vi "Trawnik.vi"() -> ()   [LabVIEW 2023]
uses:
  Trawnik_zmienne.vi
panel:
  in  "Podlewaj tryb reczny 5":bool
  in  "Podlewaj tryb reczny 4":bool
  in  "Podlewaj tryb reczny 3":bool
  in  "Podlewaj tryb reczny 2":bool
  in  "Ustaw":bool
  in  "Ilosc zraszaczy":dbl
  in  "Rok":dbl
  in  "Miesiac":dbl
  in  "Dzien":dbl
  in  "Minuta":i32=2
  in  "Godzina":i32=1
  in  "Sekcja tryb reczny":dbl
  in  "Czas podlewania":dbl
  in  "Liczba sekcji":dbl=5.0
  in  "Podlewaj tryb reczny 1":bool
  in  "Podlewaj":bool
  # "Reczny"
  # "Harmonogram"
  # "Automatyczny"
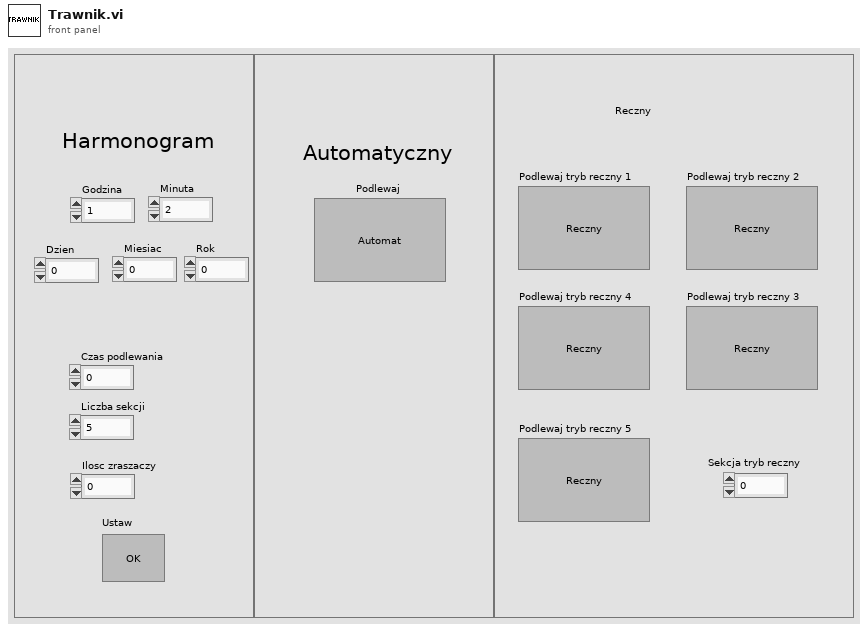
[diagram p1: front panel]
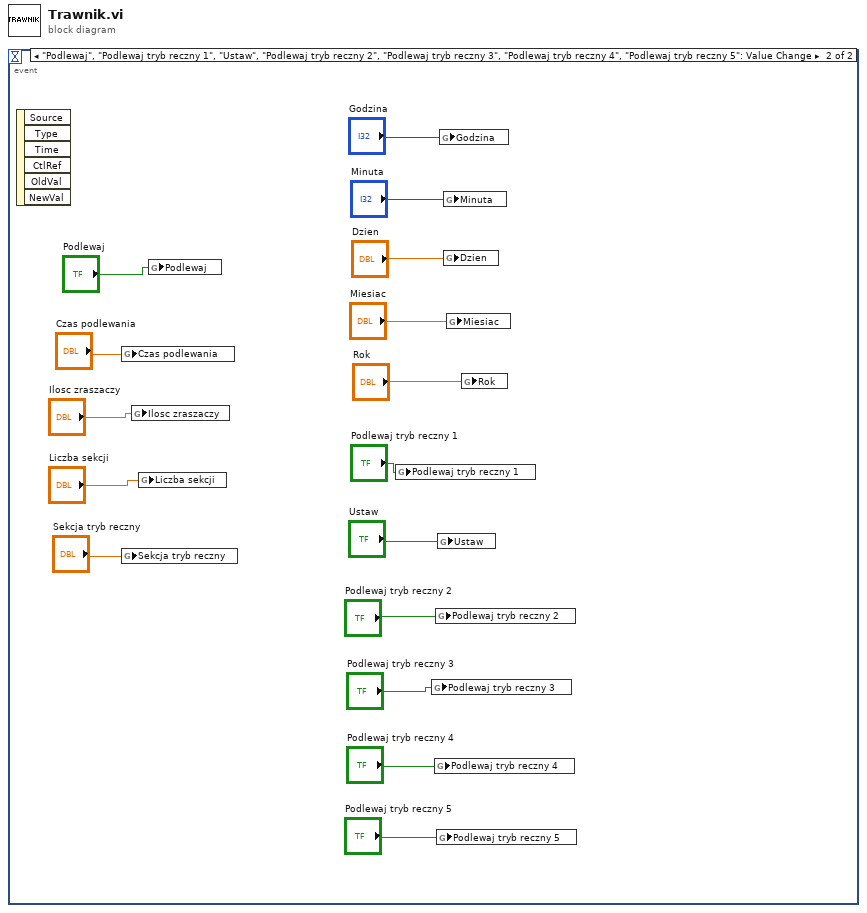
[diagram p0: block diagram]
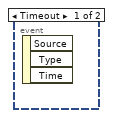
[diagram p2: hidden frame]
diagram:
  n1 = event shown="[1] \"Podlewaj\", \"Podlewaj tryb reczny 1\", \"Ustaw\", \"Podlewaj tryb reczny 2\", \"Podlewaj tryb reczny 3\", \"Podlewaj tryb reczny 4\", \"Podlewaj tryb reczny 5\": Value Change" {
    selector: _ -> [_ _]
    dyn-events: _ -> [_ _]
    timeout: _ -> [_ _]
    event Timeout {
      n2 = event-data() -> ()  [unwired: 1 in, 3 out]
    }
    event "Podlewaj", "Podlewaj tryb reczny 1", "Ustaw", "Podlewaj tryb reczny 2", "Podlewaj tryb reczny 3", "Podlewaj tryb reczny 4", "Podlewaj tryb reczny 5": Value Change {
      n3 = event-data() -> ()  [unwired: 1 in, 6 out]
      n4 = global write "Trawnik_zmienne.vi" "Czas podlewania"("Czas podlewania") -> ()
      n5 = global write "Trawnik_zmienne.vi" "Sekcja tryb reczny"("Sekcja tryb reczny") -> ()
      n6 = global write "Trawnik_zmienne.vi" "Ilosc zraszaczy"("Ilosc zraszaczy") -> ()
      n7 = global write "Trawnik_zmienne.vi" "Liczba sekcji"("Liczba sekcji") -> ()
      n8 = global write "Trawnik_zmienne.vi" "Podlewaj"("Podlewaj") -> ()
      n9 = global write "Trawnik_zmienne.vi" "Podlewaj tryb reczny 1"("Podlewaj tryb reczny 1") -> ()
      n10 = global write "Trawnik_zmienne.vi" "Podlewaj tryb reczny 3"("Podlewaj tryb reczny 3") -> ()
      n11 = global write "Trawnik_zmienne.vi" "Podlewaj tryb reczny 4"("Podlewaj tryb reczny 4") -> ()
      n12 = global write "Trawnik_zmienne.vi" "Podlewaj tryb reczny 2"("Podlewaj tryb reczny 2") -> ()
      n13 = global write "Trawnik_zmienne.vi" "Podlewaj tryb reczny 5"("Podlewaj tryb reczny 5") -> ()
      n14 = global write "Trawnik_zmienne.vi" "Ustaw"("Ustaw") -> ()
      n15 = global write "Trawnik_zmienne.vi" "Godzina"("Godzina") -> ()
      n16 = global write "Trawnik_zmienne.vi" "Minuta"("Minuta") -> ()
      n17 = global write "Trawnik_zmienne.vi" "Dzien"("Dzien") -> ()
      n18 = global write "Trawnik_zmienne.vi" "Miesiac"("Miesiac") -> ()
      n19 = global write "Trawnik_zmienne.vi" "Rok"("Rok") -> ()
    }
  }
